vi "Read U32.vi"(7 "key":string, 8 "error in (no error)":errorcluster, 9 "default value":u32, 11 "Configuration File In":refnum<class "Configuration File.lvclass">) -> (0 "error out":errorcluster, 1 "value":u32, 3 "Configuration File Out":refnum<class "Configuration File.lvclass">)   [LabVIEW 2020, in "Configuration File.lvclass"]
doc: "High-level function for reading configuration file data from process class. If the specified key is not present, it is added with the configured default value."
uses:
  Configuration File.lvclass
  C:/Git/astemes-triarc-framework/source/Framework/Configuration/Configuration.lvclass
  Base/Base.lvclass/Base.ctl
  Base/Public/Read Base Name.vi
  Private/Read Config File Ref.vi
  Configuration/Protected/Get Config Ref.vi
  <vilib>/Utility/error.llb/Clear Errors.vi
  Process/Public/Read Name.vi
  <vilib>/Utility/config.llb/Not A Config Data Refnum.vi
  <vilib>/Utility/config.llb/Read Key (U32).vi
  <vilib>/Utility/config.llb/Write Key (U32).vi
  Process/Process.lvclass
  Base/Base.lvclass
  <vilib>/Utility/config.llb/NI_LVConfig.lvlib
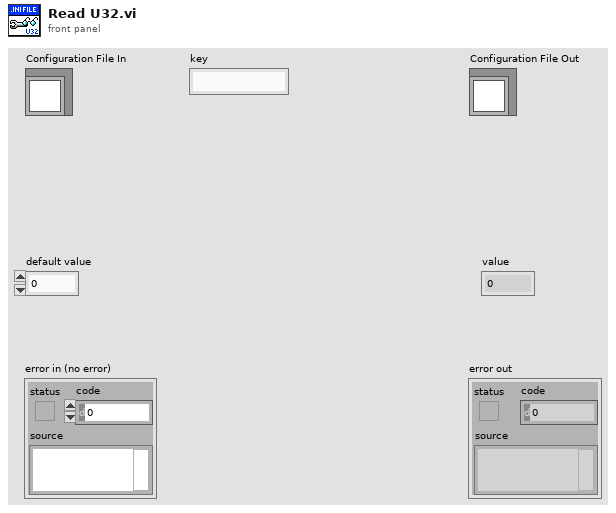
[diagram p1: front panel]
types:
  T1 = typedef "NI_LVConfig.lvlib/Config Data RefNum.ctl" = refnum<k1>
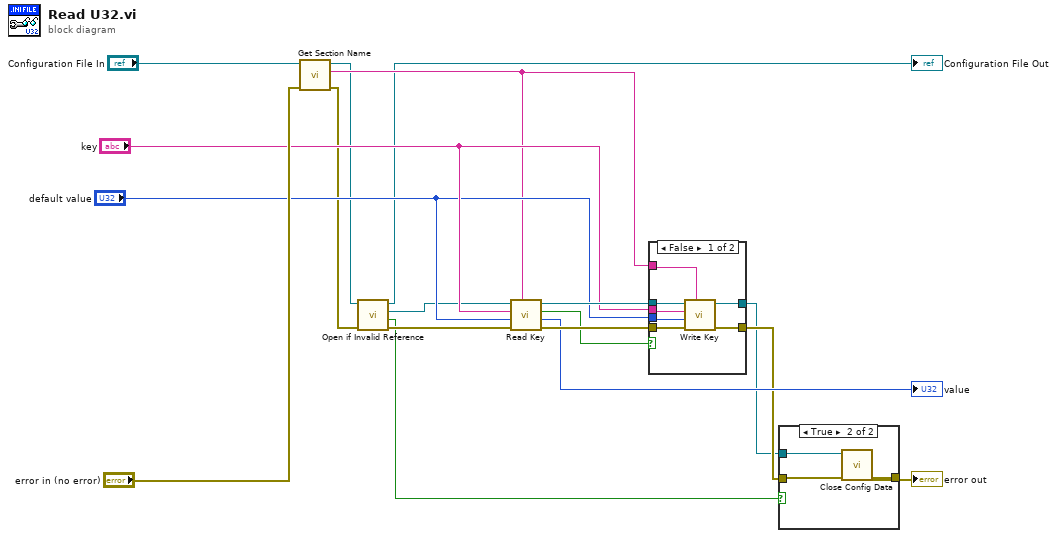
[diagram p0: block diagram]
diagram:
  n1 = call "Get Section Name.vi"("error in (no error)"="error in (no error)", "Configuration File In"="Configuration File In") -> ("error out"=w7:errorcluster, "Section Name"=w11:string, "Configuration File Out"=w9:refnum<class "Configuration File.lvclass">)  [unwired: 7 in]
  n2 = call "Open if Invalid Reference.vi"("error in (no error)"=w7, "Configuration File In"=w9) -> ("error out"=w6:errorcluster, "File opened?"=w1:bool, "refnum out"=w5:T1, "Configuration File Out"=→"Configuration File Out":refnum<class "Configuration File.lvclass">)  [unwired: 6 in]
  n3 = call-poly <vilib>:"Read Key.vi"("section"=w11, "error in (no error)"=w6, "default value"="default value", "key"="key", "refnum"=w5) -> ("error out"=w15:errorcluster, "value"=→"value":u32, "found?"=w14:bool, "refnum out"=w16:T1)  [unwired: 3 in]
  n4 = case shown="False" w14 {
    tunnel: w16 -> [w25 w27]
    tunnel: w15 -> [w24 w26]
    tunnel: [w23 w27] -> w2
    tunnel: [w22 w26] -> w3
    tunnel: "key" -> [w21 _]
    tunnel: "default value" -> [w20 _]
    tunnel: w11 -> [w19 _]
    frame False {
      n5 = call-poly <vilib>:"Write Key.vi"("section"=w19, "error in (no error)"=w24, "value"=w20, "key"=w21, "refnum"=w25) -> ("error out"=w22:errorcluster, "refnum out"=w23:T1)  [unwired: 4 in, 1 out]
    }
    frame True {
    }
  }
  n6 = case shown="True" w1 {
    tunnel: w2 -> [_ w31]
    tunnel: w3 -> [w28 w30]
    tunnel: [w28 w29] -> w4
    frame False {
    }
    frame True {
      n7 = call <vilib>:"Close Config Data.vi"("error in (no error)"=w30, "refnum"=w31) -> ("error out"=w29:errorcluster)  [unwired: 8 in, 1 out]
    }
  }
  "error out" <- w4
